vi "SW_Gen_Draw_numbers_and_highllights.vi"(5 "Regions to mark selected":u16[](array[numeric]), 6 "Colors cluster":T1, 7 "Regions to mark set":u16[](array[numeric]), 8 "Input cluster of parameters":T2={"Amount of border segments"=8, "Border segments starting angle"=0, "Amount of midfield segments"=4, "Midfield segments starting angle"=0, "Midfield segments outer radius, mm"=60, "Amount of central segments"=1, "Center segment outer radius, mm"=30, "Diameter of the cage, mm"=180, "R-gap between segments, mm"=10} {"Diameter of the cage, mm" scale=20.0..250.0}, 9 "Cluster of image geometrical and scaling parameters":T3, 10 "Bounding rectangles":T4, 11 "Zones layout input":picture) -> (2 "Array of the segment to color correspondences":u32[][](array[numeric]), 3 "Zones layout output":picture)   [LabVIEW 2018, in "Tracker.lvlib"]
uses:
  Tracker.lvlib
panel:
  in  "Bigger bubble radius":i32=15
  in  "Bubble radius":i16=11
  in  "Font size":i16=18
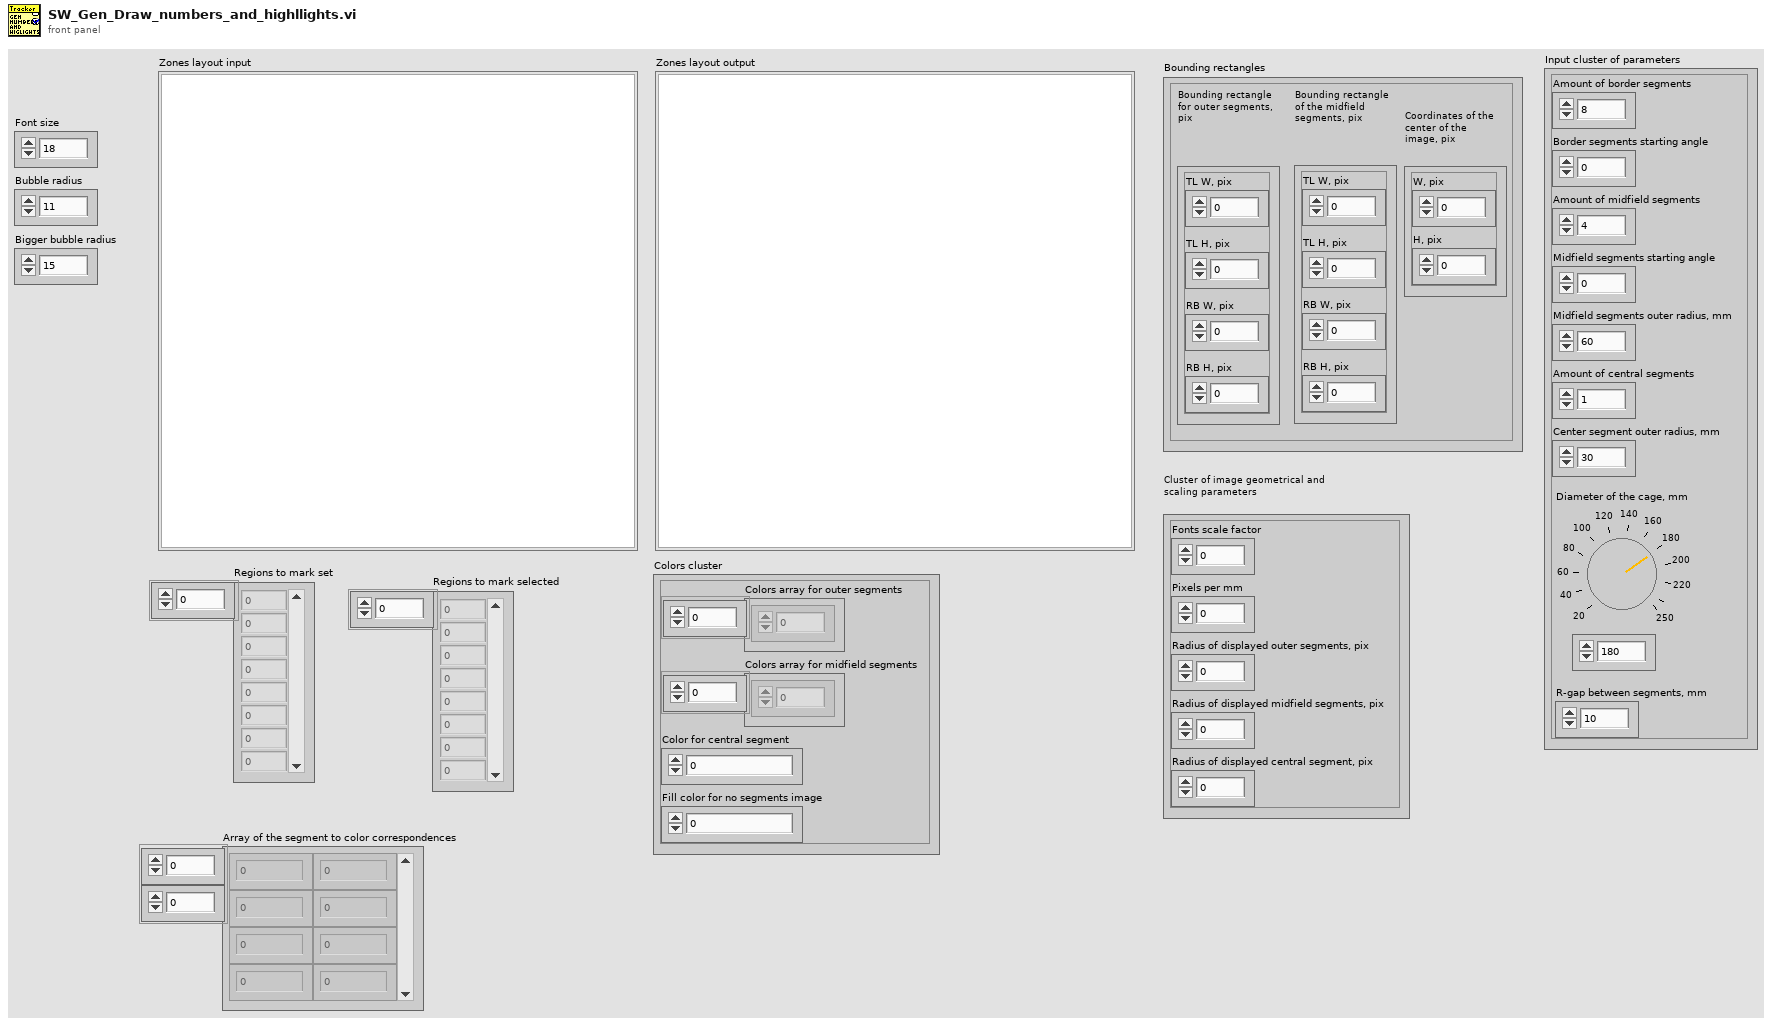
[diagram p1: front panel]
types:
  T1 = cluster{"Colors array for outer segments":u32[], "Colors array for midfield segments":u32[], "Color for central segment":u32, "Fill color for no segments image":u32}
  T2 = cluster{"Amount of border segments":u8, "Border segments starting angle":i16, "Amount of midfield segments":u8, "Midfield segments starting angle":i16, "Midfield segments outer radius, mm":u16, "Amount of central segments":u8, "Center segment outer radius, mm":u16, "Diameter of the cage, mm":u16, "R-gap between segments, mm":u8}
  T3 = cluster{"Fonts scale factor":dbl, "Pixels per mm":dbl, "Radius of displayed outer segments, pix":dbl, "Radius of displayed midfield segments, pix":dbl, "Radius of displayed central segment, pix":dbl}
  T4 = cluster{"Bounding rectangle for outer segments, pix":cluster{"TL W, pix":dbl, "TL H, pix":dbl, "RB W, pix":dbl, "RB H, pix":dbl}, "Bounding rectangle of the midfield segments, pix":cluster{"TL W, pix":dbl, "TL H, pix":dbl, "RB W, pix":dbl, "RB H, pix":dbl}, "Coordinates of the center of the image, pix":cluster{"W, pix":dbl, "H, pix":dbl}}
  T5 = enum16{"User-specified Font", "Application Font", "System Font", "Dialog Font"}
  T6 = cluster{"horizontal":enum16{"left", "center", "right"}, "vertical":enum16{"top", "center", "bottom"}}
  T7 = cluster{"TL W, pix":dbl, "TL H, pix":dbl, "RB W, pix":dbl, "RB H, pix":dbl}
  T8 = cluster{"Font Name:":string, "Size":i16, "Strikeout?":bool, "Italic?":bool, "Underline?":bool, "Outline?":bool, "Shadow?":bool, "Bold?":bool}
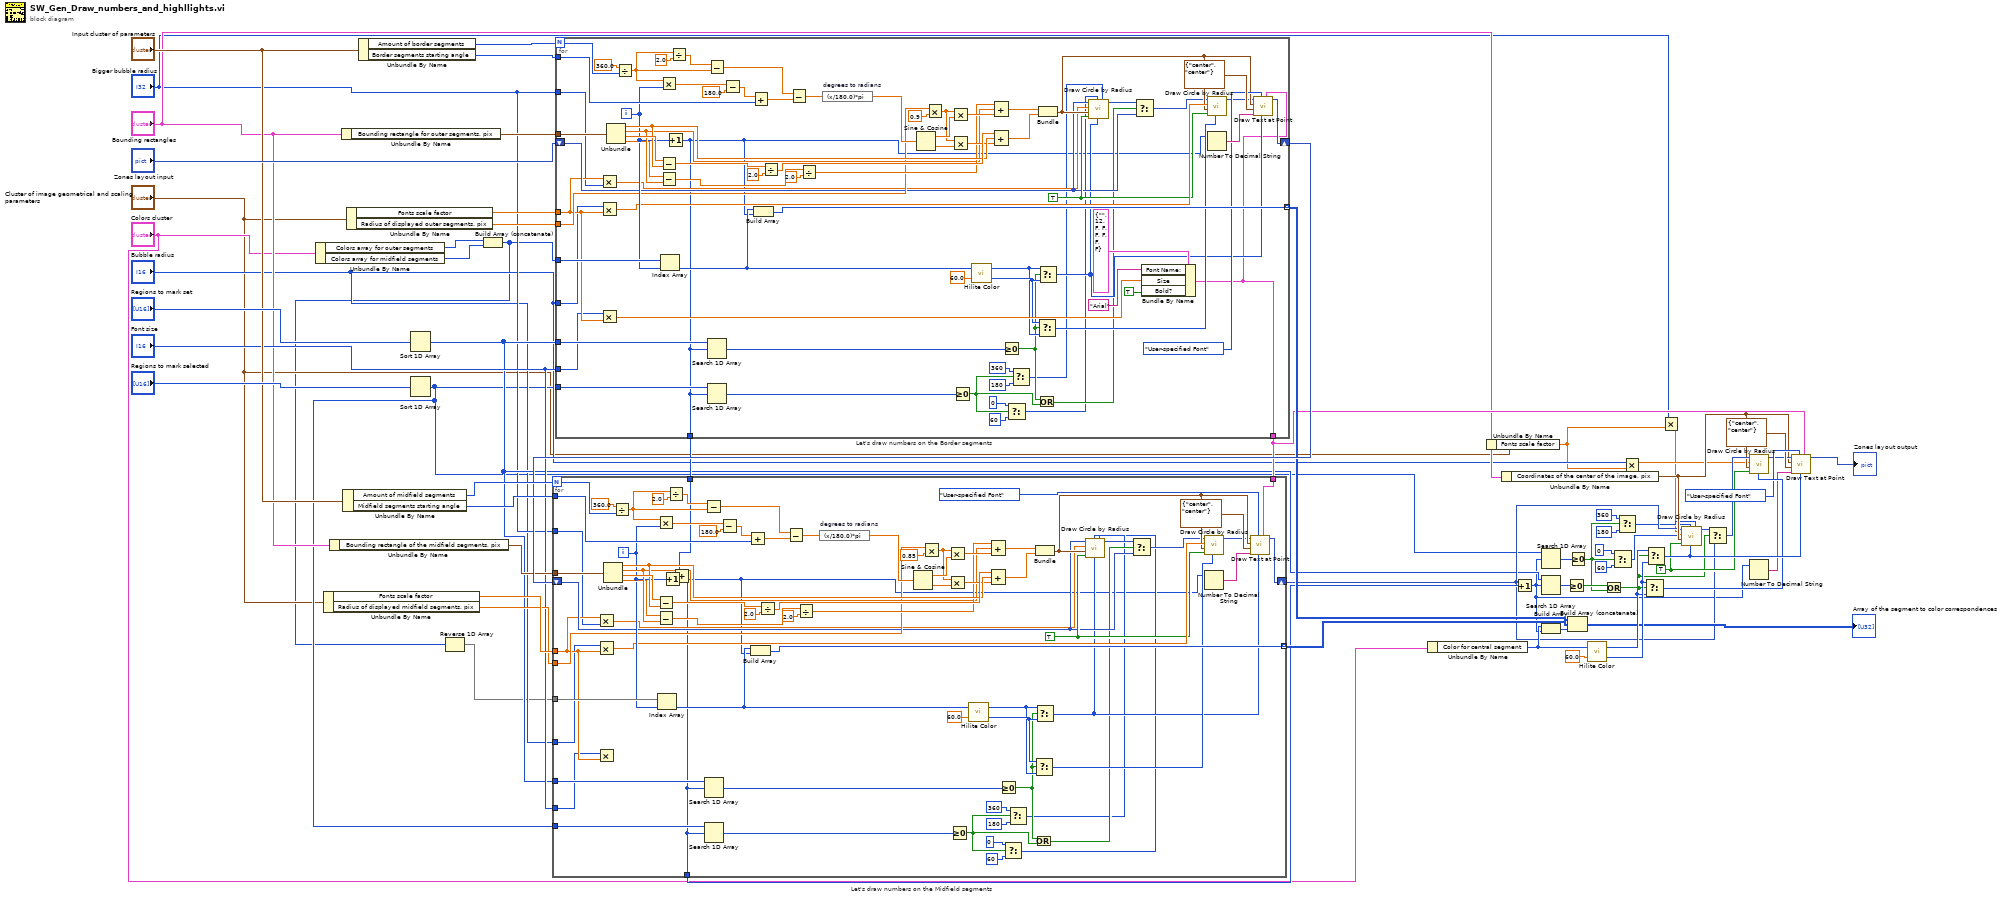
[diagram p0: block diagram]
diagram:
  w43 = TRUE ("fill?(F)")
  n1 = Unbundle By Name("Colors cluster") -> ("Colors array for outer segments"=w4:u32[], "Colors array for midfield segments"=w3:u32[])
  n2 = Unbundle By Name("Cluster of image geometrical and scaling parameters") -> ("Fonts scale factor"=w52:dbl, "Radius of displayed midfield segments, pix"=w51:dbl)
  n3 = Unbundle By Name("Bounding rectangles") -> ("Bounding rectangle of the midfield segments, pix"=w53:T7)
  n4 = Unbundle By Name("Bounding rectangles") -> ("Bounding rectangle for outer segments, pix"=w62:T7)
  n5 = Unbundle By Name("Input cluster of parameters") -> ("Amount of midfield segments"=w56:u8, "Midfield segments starting angle"=w55:i16)
  n6 = Unbundle By Name("Cluster of image geometrical and scaling parameters") -> ("Fonts scale factor"=w60:dbl, "Radius of displayed outer segments, pix"=w61:dbl)
  n7 = Unbundle By Name("Input cluster of parameters") -> ("Amount of border segments"=w59:u8, "Border segments starting angle"=w58:i16)
  n8 = Sort 1D Array(array="Regions to mark set") -> (sorted array=w22:u16[])
  n9 = Sort 1D Array(array="Regions to mark selected") -> (sorted array=w18:u16[])
  n10 = Build Array (concatenate)(w4, w3) -> (w2:u32[])
  n11 = Reverse 1D Array(array=w2) -> (reversed array=w1:u32[])
  n12 = for "Let's draw numbers on the Border segments" {
    N: w59 -> [w140]
    tunnel: w58 -> [w141]
    shift-right: [w120] -> w54
    shift-left: "Zones layout input" -> [w89]
    tunnel: w62 -> [w135]
    tunnel: w2 -> [w109]
    tunnel: w61 -> [w106]
    tunnel: [w103] -> w32 mode=indexing
    tunnel: w22 -> [w96]
    tunnel: w60 -> [w81]
    tunnel: w18 -> [w80]
    tunnel: "Font size" -> [w70]
    tunnel: "Bubble radius" -> [w69]
    tunnel: "Bigger bubble radius" -> [w68]
    tunnel: [w67] -> w49
    tunnel: [w66] -> w30
    i -> [w108]
    w92 = TRUE ("fill?(F)")
    n13 = Multiply(x=w81, y=w68) -> (x*y=w91:dbl)
    n14 = Multiply(x=w69, y=w81) -> (x*y=w97:dbl)
    n15 = Multiply(x=w70, y=w81) -> (x*y=w98:dbl)
    n16 = Unbundle(w135) -> ("TL W, pix"=w129:dbl, "TL H, pix"=w122:dbl, "RB W, pix"=w134:dbl, "RB H, pix"=w121:dbl)
    n17 = Divide(x=360.0, y=w140) -> (x/y=w110:dbl)
    n18 = Multiply(x=w110, y=w108) -> (x*y=w114:dbl)
    n19 = Subtract(x=w134, y=w129) -> (x-y=w132:dbl)
    n20 = Subtract(x=w121, y=w122) -> (x-y=w124:dbl)
    n21 = Index Array(array=w109, index=w108) -> (element=w86:u32)
    n22 = Increment(x=w108) -> (x+1=w67:i32)
    n23 = Divide(x=w110, y=2.0) -> (x/y=w112:dbl)
    n24 = Subtract(x=w112, y=w110) -> (x-y=w111:dbl)
    n25 = Search 1D Array(1D array=w96, element=w67) -> (index of element=w95:i32)  [unwired: 1 in]
    n26 = Search 1D Array(1D array=w80, element=w67) -> (index of element=w79:i32)  [unwired: 1 in]
    n27 = Subtract(x=w114, y=180.0) -> (x-y=w115:dbl)
    n28 = Add(x=w115, y=w141) -> (x+y=w138:dbl)
    n29 = Build Array(w86, w67) -> (w103:u32[])
    n30 = Divide(x=w132, y=2.0) -> (x/y=w130:dbl)
    n31 = Subtract(x=w111, y=w138) -> (x-y=w137:dbl)
    n32 = Divide(x=w124, y=2.0) -> (x/y=w126:dbl)
    n33 = expression code="(x/180.0)*pi" "degrees to radians"(w137) -> (w136:dbl)
    n34 = Sine & Cosine(0:w136) -> (1:w123:dbl, 2:w133:dbl)
    n35 = Multiply(x=w106, y=0.9) -> (x*y=w105:dbl)
    n36 = Multiply(x=w105, y=w123) -> (x*y=w127:dbl)
    n37 = Multiply(x=w105, y=w133) -> (x*y=w128:dbl)
    n38 = Greater Or Equal To 0?(x=w79) -> (x >= 0?=w72:bool)
    n39 = call <vilib>:"Hilite Color.vi"("Percentage(30)"=60.0, "Color In"=w86) -> ("Shadow"=w85:u32, "Hilite"=w84:u32)
    n40 = Compound Arithmetic op=ADD(w126, w122, w127) -> (w116:dbl)
    n41 = Compound Arithmetic op=ADD(w130, w129, w128) -> (w117:dbl)
    n42 = Greater Or Equal To 0?(x=w95) -> (x >= 0?=w83:bool)
    n43 = Select(t=i16 0 ("t 2"), s=w72, f=i16 60 ("start angle(0)")) -> (s? t:f=w73:i16)
    n44 = Select(t=i16 360, s=w72, f=i16 180 ("arc size(360)")) -> (s? t:f=w76:i16)
    n45 = Or(x=w83, y=w72) -> (x .or. y?=w77:bool)
    n46 = Select(t=w85, s=w83, f=w84) -> (s? t:f=w82:u32)
    n47 = Bundle(w116, w117) -> (w93:cluster{dbl, dbl})  [unwired: 1 in]
    n48 = Select(t=w84, s=w83, f=w85) -> (s? t:f=w78:u32)
    n49 = call <vilib>:"Draw Circle by Radius.vi"("arc size(360)"=w76, "color(black)"=w78, "start angle(0)"=w73, "fill?(F)"=w92, "pixel center"=w93, "radius"=w91, "picture"=w89) -> ("new picture"=w94:picture)  [unwired: 4 in]
    n50 = Select(t=w94, s=w77, f=w89) -> (s? t:f=w88:picture)
    n51 = Bundle By Name(cluster=T8 {"Font Name:"="", "Size"=12, "Strikeout?"=FALSE, "Italic?"=FALSE, "Underline?"=FALSE, "Outline?"=FALSE, "Shadow?"=FALSE, "Bold?"=FALSE} ("[user-specified font]"), "Font Name:"="Arial", "Size"=w98, "Bold?"=TRUE) -> (w66:T8)
    n52 = call <vilib>:"Draw Circle by Radius.vi"("color(black)"=w82, "fill?(F)"=w92, "pixel center"=w93, "radius"=w97, "picture"=w88) -> ("new picture"=w87:picture)  [unwired: 6 in]
    n53 = Number To Decimal String(number=w67) -> (decimal integer string=w118:string)  [unwired: 1 in]
    n54 = call <vilib>:"Draw Text at Point.vi"("[user-specified font]"=w66, "text color(black)"=w78, "desired font(Application)"=T5."User-specified Font", "text"=w118, "alignment(left, top)"=T6 {"horizontal"=enum."center", "vertical"=enum."center"}, "origin"=w93, "picture"=w87) -> ("new picture"=w120:picture)  [unwired: 3 in, 1 out]
  }
  n55 = for "Let's draw numbers on the Midfield segments" {
    N: w56 -> [w215]
    tunnel: w55 -> [w216]
    shift-right: [w195] -> w23
    shift-left: w54 -> [w168]
    tunnel: w53 -> [w210]
    tunnel: w1 -> [w184]
    tunnel: w51 -> [w181]
    tunnel: [w178] -> w31 mode=indexing
    tunnel: w22 -> [w175]
    tunnel: w52 -> [w160]
    tunnel: w18 -> [w158]
    tunnel: "Font size" -> [w148]
    tunnel: "Bubble radius" -> [w147]
    tunnel: "Bigger bubble radius" -> [w146]
    tunnel: w49 -> [w145]
    tunnel: w30 -> [w144]
    tunnel: [w143] -> w29
    i -> [w183]
    w171 = TRUE ("fill?(F)")
    n56 = Multiply(x=w160, y=w146) -> (x*y=w170:dbl)
    n57 = Multiply(x=w147, y=w160) -> (x*y=w176:dbl)
    n58 = Multiply(x=w148, y=w160) -> ()  [unwired: 1 out]
    n59 = Unbundle(w210) -> ("TL W, pix"=w204:dbl, "TL H, pix"=w197:dbl, "RB W, pix"=w209:dbl, "RB H, pix"=w196:dbl)
    n60 = Divide(x=360.0, y=w215) -> (x/y=w185:dbl)
    n61 = Multiply(x=w185, y=w183) -> (x*y=w189:dbl)
    n62 = Subtract(x=w209, y=w204) -> (x-y=w207:dbl)
    n63 = Subtract(x=w196, y=w197) -> (x-y=w199:dbl)
    n64 = Index Array(array=w184, index=w183) -> (element=w165:u32)
    n65 = Increment(x=w183) -> (x+1=w159:i32)
    n66 = Divide(x=w185, y=2.0) -> (x/y=w187:dbl)
    n67 = Add(x=w145, y=w159) -> (x+y=w143:i32)
    n68 = Subtract(x=w187, y=w185) -> (x-y=w186:dbl)
    n69 = Search 1D Array(1D array=w175, element=w143) -> (index of element=w174:i32)  [unwired: 1 in]
    n70 = Search 1D Array(1D array=w158, element=w143) -> (index of element=w157:i32)  [unwired: 1 in]
    n71 = Subtract(x=w189, y=180.0) -> (x-y=w190:dbl)
    n72 = Add(x=w190, y=w216) -> (x+y=w213:dbl)
    n73 = Build Array(w165, w143) -> (w178:u32[])
    n74 = Divide(x=w207, y=2.0) -> (x/y=w205:dbl)
    n75 = Subtract(x=w186, y=w213) -> (x-y=w212:dbl)
    n76 = Divide(x=w199, y=2.0) -> (x/y=w201:dbl)
    n77 = expression code="(x/180.0)*pi" "degrees to radians"(w212) -> (w211:dbl)
    n78 = Sine & Cosine(0:w211) -> (1:w198:dbl, 2:w208:dbl)
    n79 = Multiply(x=w181, y=0.85) -> (x*y=w180:dbl)
    n80 = Multiply(x=w180, y=w198) -> (x*y=w202:dbl)
    n81 = Multiply(x=w180, y=w208) -> (x*y=w203:dbl)
    n82 = Greater Or Equal To 0?(x=w157) -> (x >= 0?=w150:bool)
    n83 = call <vilib>:"Hilite Color.vi"("Percentage(30)"=60.0, "Color In"=w165) -> ("Shadow"=w164:u32, "Hilite"=w163:u32)
    n84 = Compound Arithmetic op=ADD(w201, w197, w202) -> (w191:dbl)
    n85 = Compound Arithmetic op=ADD(w205, w204, w203) -> (w192:dbl)
    n86 = Greater Or Equal To 0?(x=w174) -> (x >= 0?=w162:bool)
    n87 = Select(t=i16 0 ("t 2"), s=w150, f=i16 60 ("start angle(0)")) -> (s? t:f=w151:i16)
    n88 = Select(t=i16 360, s=w150, f=i16 180 ("arc size(360)")) -> (s? t:f=w154:i16)
    n89 = Or(x=w162, y=w150) -> (x .or. y?=w155:bool)
    n90 = Select(t=w164, s=w162, f=w163) -> (s? t:f=w161:u32)
    n91 = Bundle(w191, w192) -> (w172:cluster{dbl, dbl})  [unwired: 1 in]
    n92 = Select(t=w163, s=w162, f=w164) -> (s? t:f=w156:u32)
    n93 = call <vilib>:"Draw Circle by Radius.vi"("arc size(360)"=w154, "color(black)"=w156, "start angle(0)"=w151, "fill?(F)"=w171, "pixel center"=w172, "radius"=w170, "picture"=w168) -> ("new picture"=w173:picture)  [unwired: 4 in]
    n94 = Select(t=w173, s=w155, f=w168) -> (s? t:f=w167:picture)
    n95 = call <vilib>:"Draw Circle by Radius.vi"("color(black)"=w161, "fill?(F)"=w171, "pixel center"=w172, "radius"=w176, "picture"=w167) -> ("new picture"=w166:picture)  [unwired: 6 in]
    n96 = Number To Decimal String(number=w143) -> (decimal integer string=w193:string)  [unwired: 1 in]
    n97 = call <vilib>:"Draw Text at Point.vi"("[user-specified font]"=w144, "text color(black)"=w156, "desired font(Application)"=T5."User-specified Font", "text"=w193, "alignment(left, top)"=T6 {"horizontal"=enum."center", "vertical"=enum."center"}, "origin"=w172, "picture"=w166) -> ("new picture"=w195:picture)  [unwired: 3 in, 1 out]
  }
  n98 = Unbundle By Name("Colors cluster") -> ("Color for central segment"=w25:u32)
  n99 = Unbundle By Name("Cluster of image geometrical and scaling parameters") -> ("Fonts scale factor"=w5:dbl)
  n100 = Unbundle By Name("Bounding rectangles") -> ("Coordinates of the center of the image, pix"=w27:cluster{"W, pix":dbl, "H, pix":dbl})
  n101 = Increment(x=w29) -> (x+1=w17:i32)
  n102 = Search 1D Array(1D array=w18, element=w17) -> (index of element=w19:i32)  [unwired: 1 in]
  n103 = Search 1D Array(1D array=w22, element=w17) -> (index of element=w41:i32)  [unwired: 1 in]
  n104 = Build Array(w25, w17) -> (w37:u32[])
  n105 = Greater Or Equal To 0?(x=w41) -> (x >= 0?=w46:bool)
  n106 = Build Array (concatenate)(w32, w31, w37) -> (→"Array of the segment to color correspondences":u32[][])
  n107 = Greater Or Equal To 0?(x=w19) -> (x >= 0?=w11:bool)
  n108 = call <vilib>:"Hilite Color.vi"("Percentage(30)"=60.0, "Color In"=w25) -> ("Shadow"=w45:u32, "Hilite"=w44:u32)
  n109 = Or(x=w46, y=w11) -> (x .or. y?=w16:bool)
  n110 = Select(t=i16 0 ("t 2"), s=w11, f=i16 60 ("start angle(0)")) -> (s? t:f=w9:i16)
  n111 = Select(t=i16 360, s=w11, f=i16 180 ("arc size(360)")) -> (s? t:f=w10:i16)
  n112 = Multiply(x="Bubble radius", y=w5) -> (x*y=w8:dbl)
  n113 = Select(t=w45, s=w16, f=w44) -> (s? t:f=w47:u32)
  n114 = Select(t=w44, s=w16, f=w45) -> (s? t:f=w48:u32)
  n115 = Multiply(x="Bigger bubble radius", y=w5) -> (x*y=w6:dbl)
  n116 = call <vilib>:"Draw Circle by Radius.vi"("arc size(360)"=w10, "color(black)"=w48, "start angle(0)"=w9, "fill?(F)"=w43, "pixel center"=w27, "radius"=w6, "picture"=w23) -> ("new picture"=w42:picture)  [unwired: 4 in]
  n117 = Select(t=w42, s=w16, f=w23) -> (s? t:f=w40:picture)
  n118 = call <vilib>:"Draw Circle by Radius.vi"("color(black)"=w47, "fill?(F)"=w43, "pixel center"=w27, "radius"=w8, "picture"=w40) -> ("new picture"=w34:picture)  [unwired: 6 in]
  n119 = Number To Decimal String(number=w17) -> (decimal integer string=w36:string)  [unwired: 1 in]
  n120 = call <vilib>:"Draw Text at Point.vi"("[user-specified font]"=w30, "text color(black)"=w48, "desired font(Application)"=T5."User-specified Font", "text"=w36, "alignment(left, top)"=T6 {"horizontal"=enum."center", "vertical"=enum."center"}, "origin"=w27, "picture"=w34) -> ("new picture"=→"Zones layout output":picture)  [unwired: 3 in, 1 out]
